vi "getTaskByObject.vi"(10 "Task Object":refnum<class "Task.lvclass">, 11 "BuildWorker in":refnum<class "BuildWorker.lvclass">) -> (1 "index of element":i32, 2 "Task":refnum<class "Task.lvclass">, 3 "BuildWorker out":refnum<class "BuildWorker.lvclass">)   [LabVIEW 2017, in "BuildWorker.lvlib" / "BuildWorker.lvclass"]
uses:
  BuildWorker.lvclass
  Classes/Task/Task.lvclass
  BuildWorker.lvclass/BuildWorker.ctl
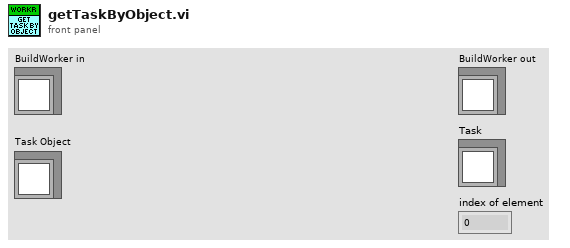
[diagram p1: front panel]
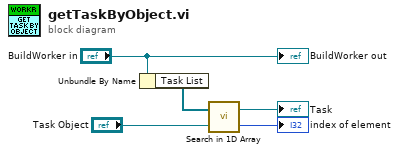
[diagram p0: block diagram]
diagram:
  n1 = Unbundle By Name("BuildWorker in") -> ("Task List"=w4:refnum<class "Task.lvclass">[])
  n2 = call "Search in 1D Array.vi"("Task in"="Task Object", "Task Array"=w4) -> ("index of element"=→"index of element":i32, "Task"=→"Task":refnum<class "Task.lvclass">)
  "BuildWorker out" <- "BuildWorker in"
